vi "ExContClns.vi"() -> ()   [LabVIEW 2010]
panel:
  in  "Software Accumulation":u32=1 min=1 step=1
  in  "Intensifier":bool
  in  "Temperature":dbl=-10.0 format="%.2f"
  in  "Exposure":dbl min=0.0 step=1e-06 format="%.5f"
  in  "stop":bool
  in  "Store":bool
  out "error out":errorcluster
  in  "error in (no error)":errorcluster
  # "ExContClns:\nThis example only works with cameras with circualar buffer capability and allow continuous clears. This vi will continuously display an image binned by 2 in both the x and the y direction. It will store in append mode the frames while the store toggle switch is on."
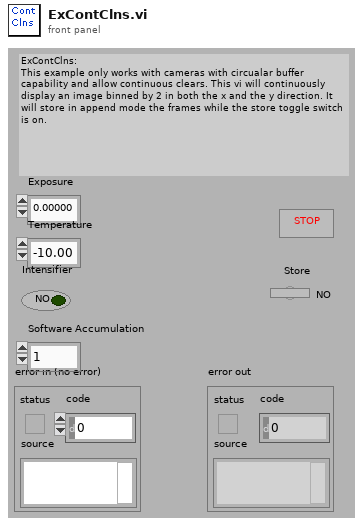
[diagram p1: front panel]
types:
  T1 = cluster{"acquire focus mode":u32, "Exposure":dbl, "Number of Images":u32, "Software Accumulation":u32}
  T2 = cluster{"Camera Handle":u32, "Pulser Handle":u32, "File Handle":u32, "Display Handle":u32, "Image Handle":u32}
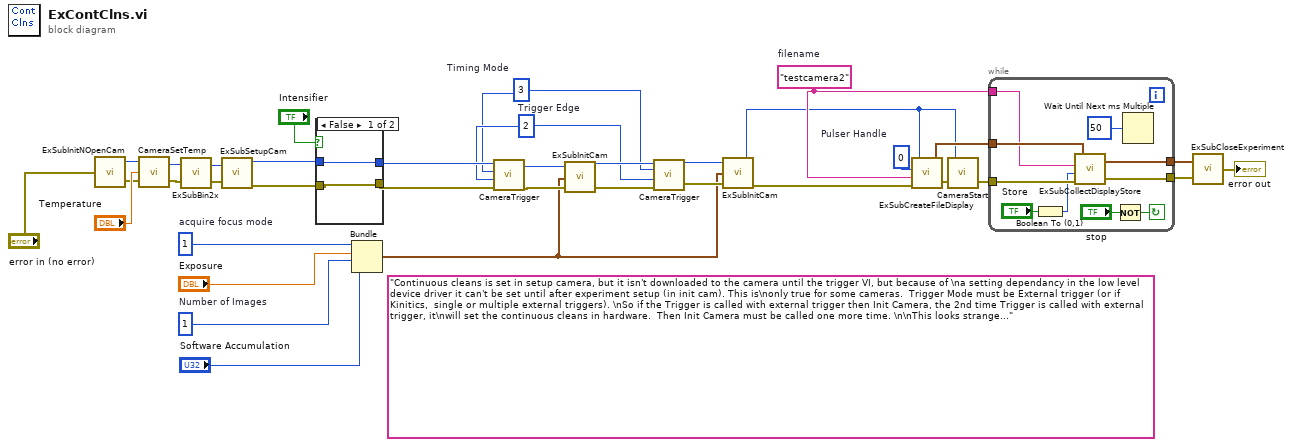
[diagram p0: block diagram]
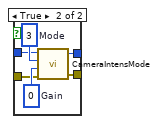
[diagram p2: hidden frame]
diagram:
  (unwired) "Continuous cleans is set in setup camera, but it isn't downloaded to the camera until the trigger VI, but because of \na setting dependancy in the low level device driver it can't be set until after experiment setup (in init cam). This is\nonly true for some cameras.  Trigger Mode must be External trigger (or if Kinitics,  single or multiple external triggers). \nSo if the Trigger is called with external trigger then Init Camera, the 2nd time Trigger is called with external trigger, it\nwill set the continuous cleans in hardware.  Then Init Camera must be called one more time. \n\nThis looks strange because the continuous cleans is set in setup camera (called before these) but it works.\nThis is due to some some idiosyncrasies in the low level camera driver."
  w1 = u32 3  # Timing Mode
  w2 = u32 2  # Trigger Edge
  w23 = u32 0  # Pulser Handle
  w25 = u32 1  # acquire focus mode
  w24 = u32 1  # Number of Images
  w36 = "testcamera2"  # filename
  n1 = call "ExSubInitNOpenCam.vi"("error in (no error)"="error in (no error)") -> ("Camera Handle"=w17:u32, "error out"=w15:errorcluster)
  n2 = call <userlib>:"CameraSetTemp.vi"("error in (no error)"=w15, "Temperature"="Temperature", "Camera Handle"=w17) -> ("error out"=w19:errorcluster, "Camera Handle"=w18:u32)
  n3 = call "ExSubBin2x.vi"("error in (no error)"=w19, "Camera Handle"=w18) -> ("error out"=w14:errorcluster, "Camera Handle"=w26:u32)
  n4 = call "ExSubSetupCam.vi"("error in (no error)"=w14, "Camera Handle"=w26) -> ("error out"=w13:errorcluster, "Camera Handle"=w12:u32)
  n5 = case shown="False" "Intensifier" {
    tunnel: [w38 w44] -> w10
    tunnel: [w37 w43] -> w11
    tunnel: w13 -> [w37 w40]
    tunnel: w12 -> [w38 w39]
    frame False {
    }
    frame True {
      w41 = u32 0  # Gain
      w42 = u32 3  # Mode
      n6 = call <userlib>:"CameraIntensMode.vi"("error in"=w40, "Intensifier Gain"=w41, "Mode"=w42, "Camera Handle"=w39) -> ("error out"=w43:errorcluster, "Camera Handle"=w44:u32)
    }
  }
  n7 = Bundle("acquire focus mode"=w25, "Exposure"="Exposure", "Number of Images"=w24, "Software Accumulation"="Software Accumulation") -> (w3:T1)  [unwired: 1 in]
  n8 = call <userlib>:"CameraTrigger.vi"("error in"=w11, "Trigger Edge"=w2, "Timing Mode"=w1, "Camera Handle"=w10) -> ("error out"=w9:errorcluster, "Camera Handle"=w8:u32)
  n9 = call "ExSubInitCam.vi"("error in (no error)"=w9, "Camera Information"=w3, "Camera Handle"=w8) -> ("error out"=w7:errorcluster, "Camera Handle"=w6:u32)
  n10 = call <userlib>:"CameraTrigger.vi"("error in"=w7, "Trigger Edge"=w2, "Timing Mode"=w1, "Camera Handle"=w6) -> ("error out"=w5:errorcluster, "Camera Handle"=w4:u32)
  n11 = call "ExSubInitCam.vi"("error in (no error)"=w5, "Camera Information"=w3, "Camera Handle"=w4) -> ("error out"=w33:errorcluster, "Camera Handle"=w22:u32)
  n12 = call "ExSubCreateFileDisplay.vi"("error in (no error)"=w33, "File and Display Name"=w36, "Pulser Handle"=w23, "Camera Handle"=w22) -> ("error out"=w27:errorcluster, "Handles Out"=w32:T2)
  n13 = call <userlib>:"CameraStart.vi"("error in"=w27, "Camera Handle"=w22) -> ("error out"=w28:errorcluster)  [unwired: 1 out]
  n14 = while {
    tunnel: w32 -> [w53]
    tunnel: w28 -> [w52]
    tunnel: w36 -> [w45]
    tunnel: [w50] -> w30
    tunnel: [w51] -> w31
    stop <- w48 continue-if-true
    n15 = Boolean To (0,1)(Boolean="Store") -> (0, 1=w46:i16)
    n16 = call "ExSubCollectDisplayStore.vi"("error in (no error)"=w52, "Store flag"=w46, "Display Title"=w45, "Handle Cluster"=w53) -> ("error out"=w50:errorcluster, "Handle Cluster Out"=w51:T2)  [unwired: 1 out]
    n17 = Not(x="stop") -> (.not. x?=w48:bool)
    n18 = Wait Until Next ms Multiple(millisecond multiple=u32 50) -> ()  [unwired: 1 out]
  }
  n19 = call "ExSubCloseExperiment.vi"("error in (no error)"=w30, "Handles In"=w31) -> ("error out"=→"error out":errorcluster)
